vi "Initialise Sinks.vi"(8 "error in (no error)":errorcluster, 11 "Logger in":refnum<class "Logger.lvclass">) -> (0 "error out":errorcluster, 3 "Logger out":refnum<class "Logger.lvclass">)   [LabVIEW 2020, in "LV Log.lvlib" / "Logger.lvclass"]
uses:
  Logger.lvclass
  Logger.lvclass/Logger.ctl
  Sinks/Sink/Sink.lvclass
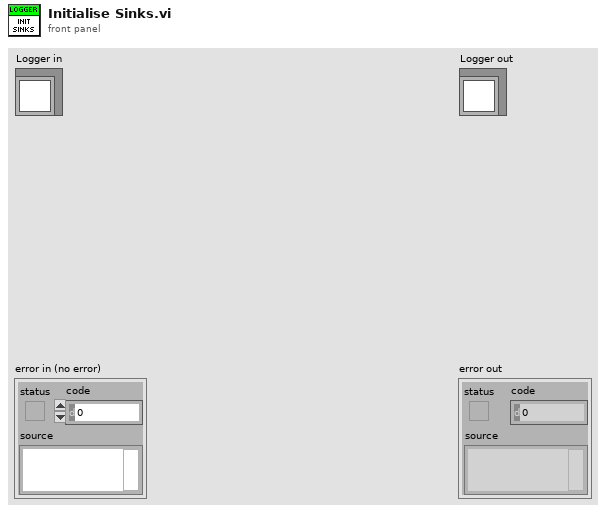
[diagram p1: front panel]
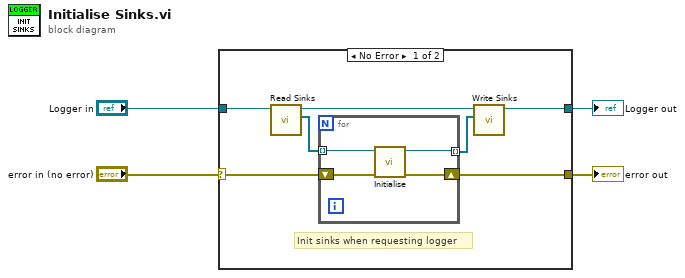
[diagram p0: block diagram]
diagram:
  n1 = case shown="No Error" "error in (no error)" {
    selector: "error in (no error)" -> [w6 w17]
    tunnel: [w5 w17] -> w3
    tunnel: [w8 w16] -> w1
    tunnel: "Logger in" -> [w7 w16]
    frame No Error {
      # "Init sinks when requesting logger"
      n2 = call "Read Sinks.vi"("Logger in"=w7) -> ("Sinks"=w11:refnum<class "Sink.lvclass">[], "Logger out"=w10:refnum<class "Logger.lvclass">)  [unwired: 8 in, 1 out]
      n3 = for {
        tunnel: w11 -> [w15] mode=indexing
        tunnel: [w14] -> w9 mode=indexing
        shift-right: [w12] -> w5
        shift-left: w6 -> [w13]
        n4 = call-dynamic "Initialise.vi"("error in (no error)"=w13, "Sink in"=w15) -> ("error out"=w12:errorcluster, "Sink out"=w14:refnum<class "Sink.lvclass">)  [unwired: 8 in]
      }
      n5 = call "Write Sinks.vi"("Sinks"=w9, "Logger in"=w10) -> ("Logger out"=w8:refnum<class "Logger.lvclass">)  [unwired: 8 in, 1 out]
    }
    frame Error {
    }
  }
  "error out" <- w3
  "Logger out" <- w1
